vi "Camera handle.vi"(0 "axis 2 (y)":dbl, 1 "axis 3 (rotation)":dbl, 2 "Center on Target":bool, 3 "View Ground":bool, 4 "Whole robot centering":bool, 7 "Stop Auto Cam movement":bool, 8 "Camera X axis center angle":i32, 9 "Seen floor angle Y":i32, 10 "Servo Get Angle X":i32, 11 "Servo Get Angle Y":i32) -> (16 "Out X [angle]":i32, 17 "Out Y [angle]":i32, 19 "Camera Centered on Target":bool)   [LabVIEW 2012]
uses:
  BotStatus.vi
panel:
  # "Angle"
  # "Angle"
  # "Angle"
  # "Angle"
  # "Valid for 3Dpro joystick\nif another joystick is used use the Y axis"
  # "Angle"
  # "Angle"
  # "Angle"
  # "Angle"
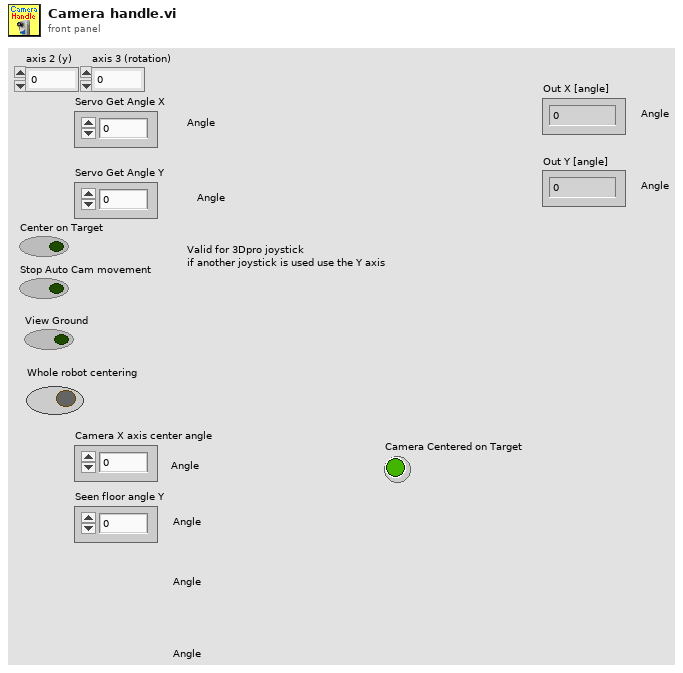
[diagram p1: front panel]
types:
  T1 = cluster{"Target Position X":dbl, "Target Position Y":dbl, "Target Found":bool}
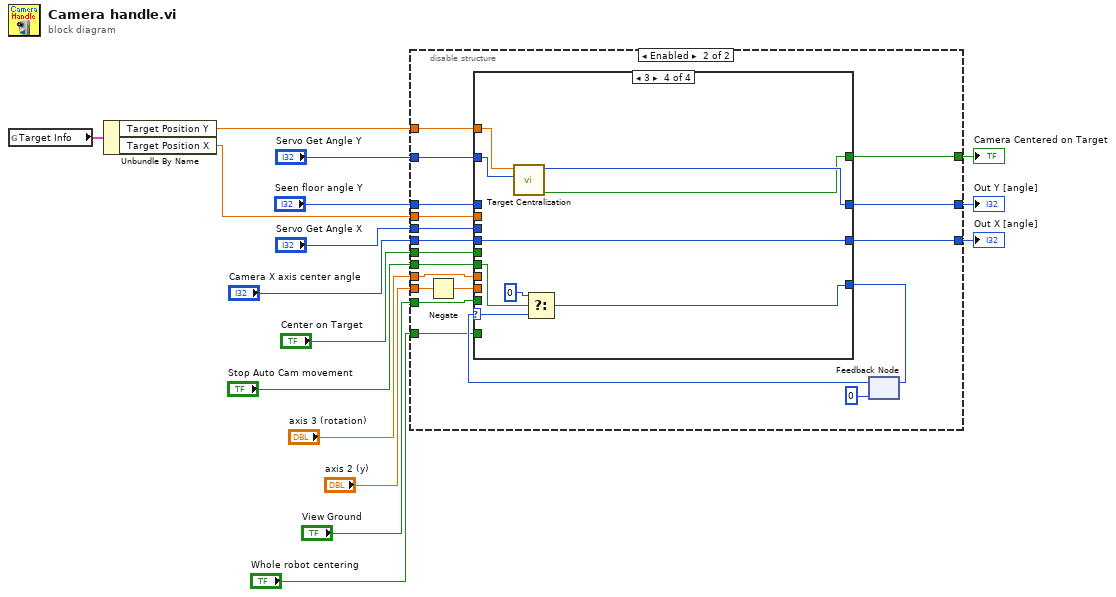
[diagram p0: block diagram]
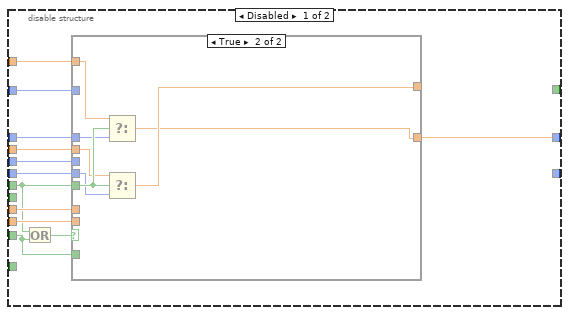
[diagram p2: hidden frame]
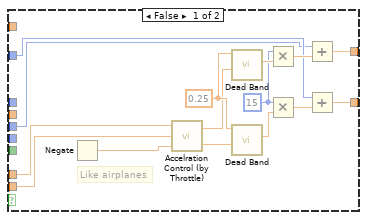
[diagram p3: hidden frame]
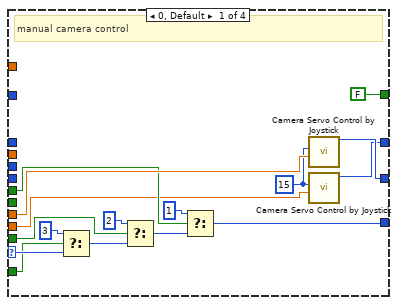
[diagram p4: hidden frame]
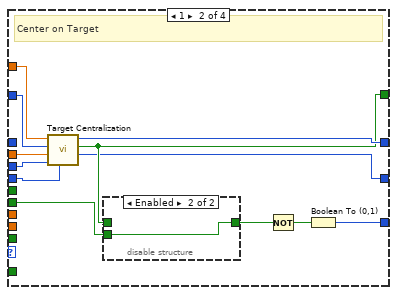
[diagram p5: hidden frame]
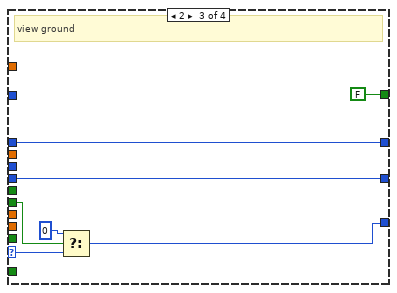
[diagram p7: hidden frame]
diagram:
  n1 = global read "BotStatus.vi" "Target Info"() -> (w5:T1)
  n2 = Unbundle By Name(w5) -> ("Target Position Y"=w4:dbl, "Target Position X"=w3:dbl)
  n3 = disable-structure shown="Enabled" {
    disable-tunnel: [w28 w68] -> w16
    disable-tunnel: "Servo Get Angle X" -> [w27 w63]
    disable-tunnel: "Servo Get Angle Y" -> [w26 w65]
    disable-tunnel: "axis 3 (rotation)" -> [w24 w64]
    disable-tunnel: "axis 2 (y)" -> [w23 w66]
    disable-tunnel: "Center on Target" -> [w22 w56]
    disable-tunnel: "View Ground" -> [w21 w55]
    disable-tunnel: "Seen floor angle Y" -> [w20 w69]
    disable-tunnel: "Camera X axis center angle" -> [w19 w70]
    disable-tunnel: w3 -> [w18 w61]
    disable-tunnel: w4 -> [w17 w62]
    disable-tunnel: [_ w60] -> w11
    disable-tunnel: "Stop Auto Cam movement" -> [_ w58]
    disable-tunnel: [_ w54] -> w2
    disable-tunnel: "Whole robot centering" -> [_ w52]
    frame Disabled {
      n4 = Or(x=w22, y=w21) -> (x .or. y?=w25:bool)
      n5 = case shown="True" w25 {
        tunnel: [w32 w51] -> w29
        tunnel: [w31 w50] -> w28
        tunnel: w27 -> [w38 _]
        tunnel: w26 -> [w39 _]
        tunnel: w24 -> [w34 _]
        tunnel: w23 -> [w33 _]
        tunnel: w22 -> [_ w49]
        tunnel: w21 -> [_ _]
        tunnel: w20 -> [_ w48]
        tunnel: w19 -> [_ w47]
        tunnel: w18 -> [_ w46]
        tunnel: w17 -> [_ w45]
        frame False {
          w37 = 15
          w44 = 0.25 ("Dead Band")
          # "Like airplanes"
          n6 = Negate() -> (-x=w30:dbl)  [unwired: 1 in]
          n7 = call "Accelration Control (by Throttle).vi"("acc"=w30, "Yinput"=w33, "Xinput"=w34) -> ("Youtput"=w35:dbl, "Xoutput"=w36:dbl)
          n8 = call "Dead Band.vi"("Axis In"=w36, "Dead Band"=w44) -> ("Axis Out"=w43:dbl)  [unwired: 9 in]
          n9 = call "Dead Band.vi"("Axis In"=w35, "Dead Band"=w44) -> ("Axis Out"=w42:dbl)  [unwired: 9 in]
          n10 = Multiply(x=w37, y=w43) -> (x*y=w40:dbl)
          n11 = Multiply(x=w37, y=w42) -> (x*y=w41:dbl)
          n12 = Add(x=w38, y=w40) -> (x+y=w32:dbl)
          n13 = Add(x=w39, y=w41) -> (x+y=w31:dbl)
        }
        frame True {
          n14 = Select(t=w45, s=w49, f=w48) -> (s? t:f=w50:dbl)
          n15 = Select(t=w46, s=w49, f=w47) -> (s? t:f=w51:dbl)
        }
      }
    }
    frame Enabled {
      n16 = Negate(x=w66) -> (-x=w67:dbl)
      n17 = feedback #1(i16 0) -> (w53:i16)
      n18 = case shown="3" w53 {
        selector: w53 -> [w72 _ w103 w109]
        tunnel: w70 -> [_ w94 w101 w116]
        tunnel: w69 -> [_ _ w106 _]
        tunnel: [w75 w93 w106 w115] -> w68
        tunnel: w67 -> [w77 _ _ _]
        tunnel: w65 -> [_ w97 _ w113]
        tunnel: w64 -> [w86 _ _ _]
        tunnel: w63 -> [_ w95 _ _]
        tunnel: w62 -> [_ w98 _ w114]
        tunnel: w61 -> [_ w96 _ _]
        tunnel: [FALSE ("centered") w90 FALSE ("centered") w112] -> w60
        tunnel: [w79 w91 w102 w110] -> w59
        tunnel: w58 -> [_ w88 w105 w108]
        tunnel: w56 -> [w81 _ _ _]
        tunnel: w55 -> [w80 _ _ _]
        tunnel: [w78 w87 w101 w116] -> w54
        tunnel: w52 -> [w71 _ _ _]
        frame 0, Default {
          w76 = 15 ("y")
          # "manual camera control"
          n19 = Select(t=i16 3, s=w71, f=w72) -> (s? t:f=w73:i16)
          n20 = Select(t=i16 2, s=w80, f=w73) -> (s? t:f=w84:i16)
          n21 = Select(t=i16 1, s=w81, f=w84) -> (s? t:f=w79:i16)
          n22 = call "Camera Servo Control by Joystick.vi"("axis control"=w86, "max jump angle"=w76) -> ("angle set"=w78:i32)  [unwired: 9 in]
          n23 = call "Camera Servo Control by Joystick.vi"("axis control"=w77, "max jump angle"=w76) -> ("angle set"=w75:i32)  [unwired: 9 in]
        }
        frame 1 {
          # "Center on Target"
          n24 = call "Target Centralization.vi"("X axis center angle"=w94, "Servo Get Angle X"=w95, "Target Position X"=w96, "Servo Get Angle Y"=w97, "Target Position Y"=w98) -> ("Servo Angle Set Point X"=w87:i32, "centered"=w90:bool, "Servo Angle Set Point Y"=w93:i32)  [unwired: 1 in, 2 out]
          n25 = disable-structure shown="Enabled" {
            disable-tunnel: [w99 w100] -> w89
            disable-tunnel: w90 -> [w99 _]
            disable-tunnel: w88 -> [_ w100]
            frame Disabled {
            }
            frame Enabled {
            }
          }
          n26 = Not(x=w89) -> (.not. x?=w92:bool)
          n27 = Boolean To (0,1)(Boolean=w92) -> (0, 1=w91:i16)
        }
        frame 2 {
          # "view ground"
          n28 = Select(t=i16 0, s=w105, f=w103) -> (s? t:f=w102:i16)
        }
        frame 3 {
          n29 = call "Target Centralization.vi"("Servo Get Angle Y"=w113, "Target Position Y"=w114) -> ("Y centerd"=w112:bool, "Servo Angle Set Point Y"=w115:i32)  [unwired: 4 in, 3 out]
          n30 = Select(t=i16 0, s=w108, f=w109) -> (s? t:f=w110:i16)
        }
      }
      n31 = feedback-in #1(w59) -> ()
    }
  }
  "Out X [angle]" <- w2
  "Out Y [angle]" <- w16
  "Camera Centered on Target" <- w11
